vi "Refresh Panel Sizes.vi"(8 "error in (no error)":errorcluster, 10 "Panels in":refnum<class "ArrayPanel.lvclass">[][](array[class]), 11 "2DArrayManager in":refnum<class "2DArrayManager.lvclass">) -> (0 "error out":errorcluster, 2 "Panels":refnum<class "ArrayPanel.lvclass">[][](array[class]), 3 "2DArrayManager out":refnum<class "2DArrayManager.lvclass">)   [LabVIEW 2020, in "OOPanel.lvlib" / "2DArrayManager.lvclass"]
uses:
  2DArrayManager.lvclass
  Desired Size.ctl
  OOPanel.lvlib
  ArrayPanel/ArrayPanel.lvclass
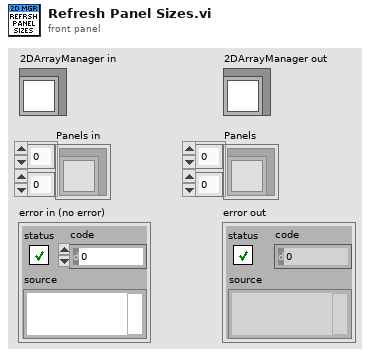
[diagram p1: front panel]
types:
  T1 = typedef "OOPanel.lvlib/Desired Size.ctl" = cluster{"Width":u32, "Height":u32}
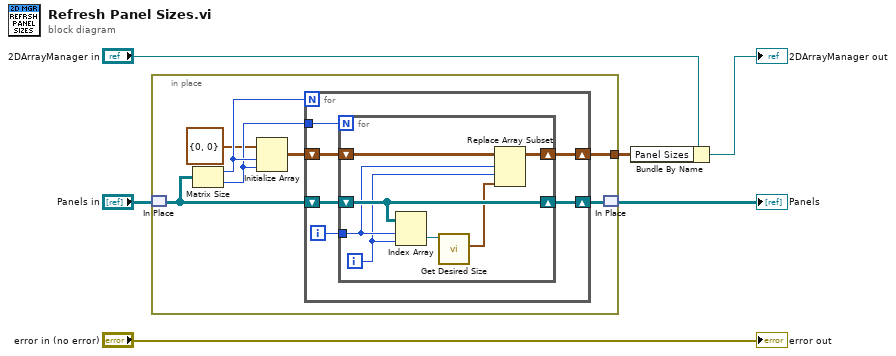
[diagram p0: block diagram]
diagram:
  n1 = in-place {
    in-place-border: [w7] -> w3
    n2 = in-place-match #1("Panels in") -> (w9:refnum<class "ArrayPanel.lvclass">[][])
    n3 = Matrix Size(0:w9) -> (1:w13:i32, 2:w12:i32)
    n4 = Initialize Array(T1 {"Width"=0, "Height"=0} ("Desired Size"), w13, w12) -> (w11:T1[][])
    n5 = for {
      N: w13 -> [_]
      tunnel: w12 -> [w19]
      shift-right: [w14] -> w7
      shift-left: w11 -> [w18]
      shift-right: [w16] -> w8
      shift-left: w9 -> [w17]
      i -> [w15]
      n6 = for {
        N: w19 -> [_]
        shift-right: [w20] -> w14
        shift-left: w18 -> [w24]
        shift-right: [w26] -> w16
        shift-left: w17 -> [w26]
        tunnel: w15 -> [w22]
        i -> [w21]
        n7 = Index Array(array=w26, index (row)=w22, index (col)=w21) -> (element=w25:refnum<class "ArrayPanel.lvclass">)
        n8 = call-dynamic "Get Desired Size.vi"("ArrayPanel in"=w25) -> ("Desired Size"=w23:T1)  [unwired: 8 in, 2 out]
        n9 = Replace Array Subset(array=w24, new element=w23, index (row)=w22, index (col)=w21) -> (w20:T1[][])
      }
    }
    n10 = in-place-match #1(w8) -> (→"Panels":refnum<class "ArrayPanel.lvclass">[][])
  }
  n11 = Bundle By Name(cluster="2DArrayManager in", "Panel Sizes"=w3) -> (→"2DArrayManager out":refnum<class "2DArrayManager.lvclass">)
  "error out" <- "error in (no error)"
